vi "fgv_RefDAQParam.vi"(8 "error in (no error)":errorcluster, 10 "Function":enum16{"Initialize", "Write", "Read"}(ring)=enum."Read", 11 "RefDAQParam in":T1={"Full Frame Size"=0, "Ref Field of View"=0.0, "Ref Zoom"=0, "Ref_dwellTime"=0.0, "Ref X-pixels-per-line(Npxr)"=0, "Ref Y-lines-per-image(Npyr)"=0, "Ref Z-lines-per-image"=0, "Ref Scan Cycles"=0, "Ref threshold"=0, "Ref average"=1, "Sliding Average"=FALSE, "proportioanl_scale"=1.5999755859375, "Integral_scale"=2047.9375, "proportioanl_scaleZ"=1.5999755859375, "Integral_scaleZ"=400.0, "Diff_threshold"=0.0, "Diff_threshold _z"=0.0, "scale"=0.0, "Control algorithm"=enum."Kalman", "New line trigger enabled"=TRUE, "Slide Averaging"=FALSE, "Ref count reset enabled"=FALSE} {"proportioanl_scaleZ" format="%#_15g"; "Diff_threshold" format="%#_15g"; "Diff_threshold _z" format="%#_15g"; "scale" format="%#_15g"; "proportioanl_scale" format="%#_15g"}) -> (0 "error out":errorcluster, 3 "RefDAQParam":T1={"Full Frame Size"=0, "Ref Field of View"=0.0, "Ref Zoom"=0, "Ref_dwellTime"=0.0, "Ref X-pixels-per-line(Npxr)"=0, "Ref Y-lines-per-image(Npyr)"=0, "Ref Z-lines-per-image"=0, "Ref Scan Cycles"=0, "Ref threshold"=0, "Ref average"=1, "Sliding Average"=FALSE, "proportioanl_scale"=1.5999755859375, "Integral_scale"=2047.9375, "proportioanl_scaleZ"=1.5999755859375, "Integral_scaleZ"=400.0, "Diff_threshold"=0.0, "Diff_threshold _z"=0.0, "scale"=0.0, "Control algorithm"=enum."Kalman", "New line trigger enabled"=TRUE, "Slide Averaging"=FALSE, "Ref count reset enabled"=FALSE} {"proportioanl_scaleZ" format="%#_15g"; "Diff_threshold" format="%#_15g"; "Diff_threshold _z" format="%#_15g"; "scale" format="%#_15g"; "proportioanl_scale" format="%#_15g"})   [LabVIEW 2017]
uses:
  Acquisition/Typedefs/Ref DAQ Param.ctl
  Movement Correction/Typedefs/Control algorithm.ctl
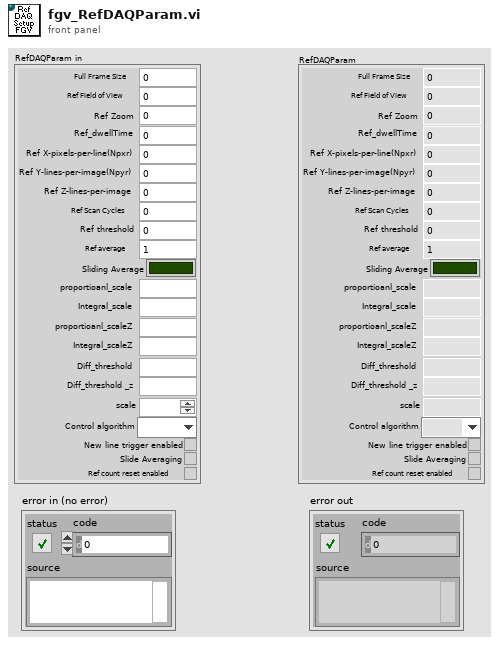
[diagram p1: front panel]
types:
  T1 = typedef "Ref DAQ Param.ctl" = cluster{"Full Frame Size":u16, "Ref Field of View":sgl, "Ref Zoom":i8, "Ref_dwellTime":sgl, "Ref X-pixels-per-line(Npxr)":i16, "Ref Y-lines-per-image(Npyr)":i16, "Ref Z-lines-per-image":i16, "Ref Scan Cycles":i32, "Ref threshold":u16, "Ref average":u16, "Sliding Average":bool, "proportioanl_scale":fxp<+,16,2>, "Integral_scale":fxp<+/-,16,12>, "proportioanl_scaleZ":fxp<+,16,2>, "Integral_scaleZ":fxp<+/-,16,12>, "Diff_threshold":fxp<+,16,2>, "Diff_threshold _z":fxp<+,16,2>, "scale":fxp<+,16,2>, "Control algorithm":T2, "New line trigger enabled":bool, "Slide Averaging":bool, "Ref count reset enabled":bool}
  T2 = typedef "Control algorithm.ctl" = enum16{"PID", "Kalman"}
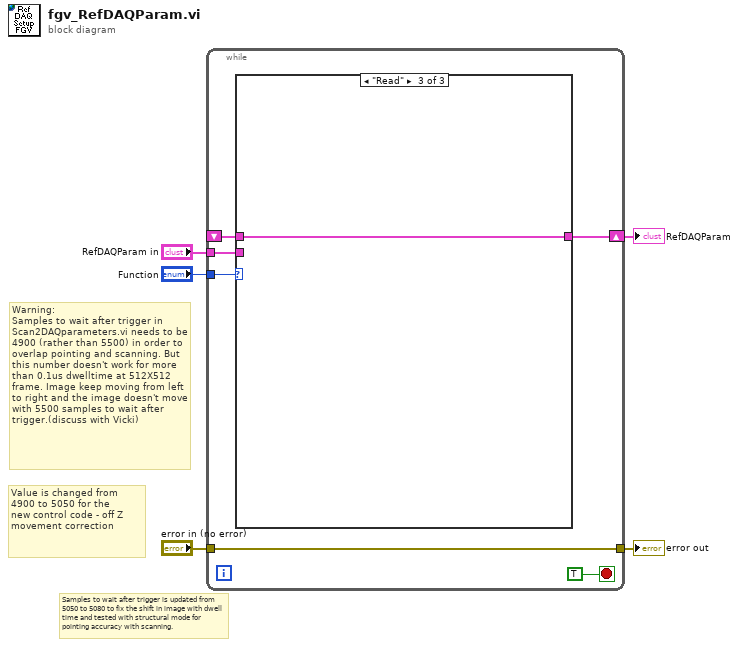
[diagram p0: block diagram]
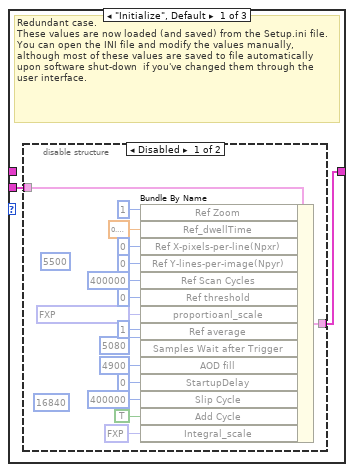
[diagram p2: hidden frame]
diagram:
  # "Samples to wait after trigger is updated from 5050 to 5080 to fix the shift in image with dwell time and tested with structural mode for pointing accuracy with scanning."
  # "Value is changed from 4900 to 5050 for the \nnew control code - off Z movement correction"
  # "Warning:\nSamples to wait after trigger in Scan2DAQparameters.vi needs to be 4900 (rather than 5500) in order to overlap pointing and scanning. But this number doesn't work for more than 0.1us dwelltime at 512X512 frame. Image keep moving from left to right and the image doesn't move with 5500 samples to wait after trigger.(discuss with Vicki)"
  n1 = while {
    tunnel: "Function" -> [w10]
    shift-right: [w9] -> w3
    shift-left: _ -> [w8]
    tunnel: "RefDAQParam in" -> [w7]
    tunnel: "error in (no error)" -> [w6]
    tunnel: [w6] -> w1
    stop <- TRUE stop-if-true
    n2 = case shown="\"Read\"" w10 {
      tunnel: [w12 w30 w31] -> w9
      tunnel: w8 -> [_ _ w31]
      tunnel: w7 -> [w13 w30 _]
      frame "Initialize", Default {
        # "Redundant case.\nThese values are now loaded (and saved) from the Setup.ini file. You can open the INI file and modify the values manually, although most of these values are saved to file automatically upon software shut-down  if you've changed them through the user interface."
        n3 = disable-structure shown="Disabled" {
          disable-tunnel: w13 -> [w29 _]
          disable-tunnel: [w28 _] -> w12
          frame Disabled {
            (unwired) u16 5500 ("Samples Wait after Trigger")
            (unwired) u32 16840 ("Slip Cycle")
            n4 = Bundle By Name(cluster=w29, "Ref Zoom"=i8 1, "Ref_dwellTime"=sgl 0.2, "Ref X-pixels-per-line(Npxr)"=i16 0, "Ref Y-lines-per-image(Npyr)"=i16 0 ("Ref Y-pixels-per-line(NPyr)"), "Ref Scan Cycles"=400000, "Ref threshold"=u16 0 ("threshold"), "proportioanl_scale"=fxp<+,16,2> 1.5999755859375, "Ref average"=u16 1 ("Average"), "Samples Wait after Trigger"=u16 5080, "AOD fill"=u16 4900, "StartupDelay"=0, "Slip Cycle"=u32 400000, "Add Cycle"=TRUE, "Integral_scale"=fxp<+/-,16,12> 450.0) -> (w28:T1)
          }
          frame Enabled {
          }
        }
      }
      frame "Write" {
      }
      frame "Read" {
      }
    }
  }
  "RefDAQParam" <- w3
  "error out" <- w1
